vi "LVFunction_Imop_SlopesPostProcessor_Apply Apply Filter.vi"(0 "HasoSlopes in":refnum<class "HasoSlopes.lvclass">, 5 "HasoSlopes OUT":refnum<class "HasoSlopes.lvclass">, 7 "filter":T1, 11 "error in (no error)":errorcluster) -> (4 "HasoSlopes out":refnum<class "HasoSlopes.lvclass">, 6 "HasoSlopes OUT 2":refnum<class "HasoSlopes.lvclass">, 15 "error out":errorcluster)   [LabVIEW 2020]
uses:
  HasoSlopes.lvclass
  SlopesPostProcessorList - Filter.ctl
  LVClass_HasoSlopes Read HasoSlopes _ property.vi
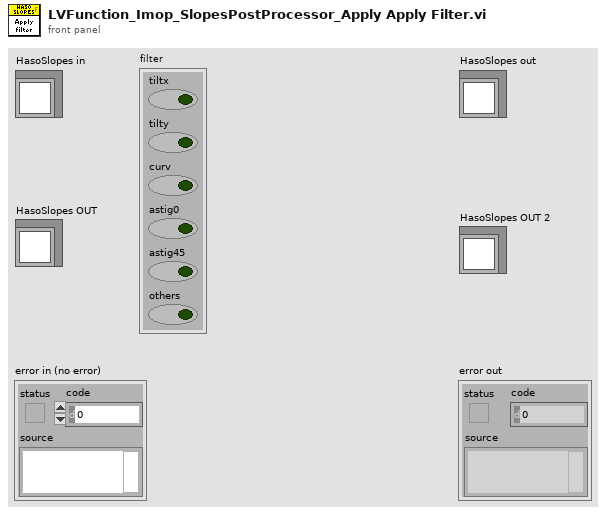
[diagram p1: front panel]
types:
  T1 = typedef "SlopesPostProcessorList - Filter.ctl" = cluster{"tiltx":bool, "tilty":bool, "curv":bool, "astig0":bool, "astig45":bool, "others":bool}
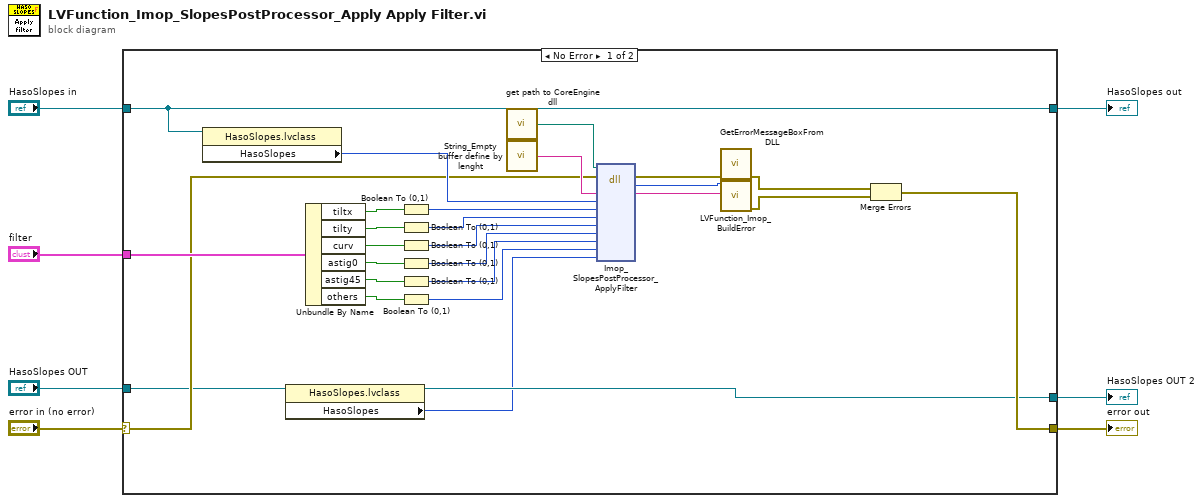
[diagram p0: block diagram]
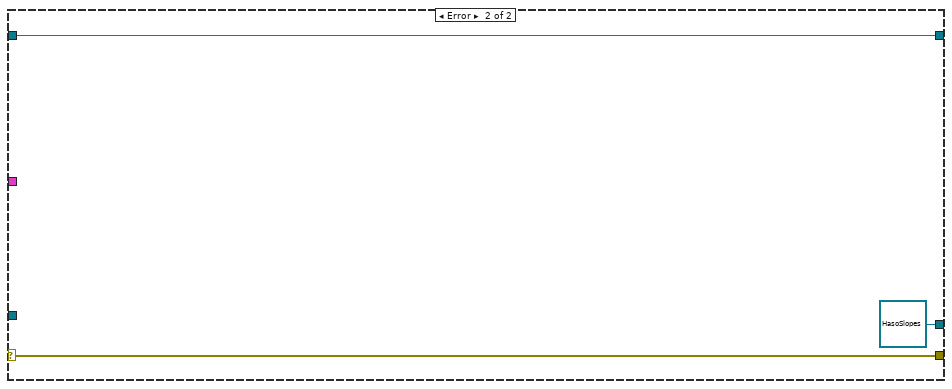
[diagram p2: hidden frame]
diagram:
  n1 = case shown="No Error" "error in (no error)" {
    selector: "error in (no error)" -> [w13 w37]
    tunnel: [w12 w37] -> w3
    tunnel: [w9 w36] -> w4
    tunnel: "HasoSlopes in" -> [w9 w36]
    tunnel: "filter" -> [w14 _]
    tunnel: "HasoSlopes OUT" -> [w11 _]
    tunnel: [w10 refnum<class "HasoSlopes.lvclass"> refnum ("HasoSlopes OUT")] -> w5
    frame No Error {
      n2 = property class="HasoSlopes.lvclass"(reference=w9) -> ("HasoSlopes"=w15:i32)  [unwired: 1 in, 2 out]
      n3 = property class="HasoSlopes.lvclass"(reference=w11) -> (reference out=w10:refnum<class "HasoSlopes.lvclass">, "HasoSlopes"=w8:i32)  [unwired: 1 in, 1 out]
      n4 = Unbundle By Name(w14) -> ("tiltx"=w23:bool, "tilty"=w24:bool, "curv"=w25:bool, "astig0"=w26:bool, "astig45"=w27:bool, "others"=w28:bool)
      n5 = Boolean To (0,1)(Boolean=w23) -> (0, 1=w29:i16)
      n6 = Boolean To (0,1)(Boolean=w24) -> (0, 1=w30:i16)
      n7 = Boolean To (0,1)(Boolean=w25) -> (0, 1=w31:i16)
      n8 = Boolean To (0,1)(Boolean=w26) -> (0, 1=w32:i16)
      n9 = Boolean To (0,1)(Boolean=w27) -> (0, 1=w33:i16)
      n10 = Boolean To (0,1)(Boolean=w28) -> (0, 1=w34:i16)
      n11 = call "get path to CoreEngine dll.vi"() -> ("path to c_interface_vc100.dll"=w16:path)  [unwired: 12 in, 3 out]
      n12 = call "String_Empty buffer define by lenght.vi"() -> ("Empty buffer"=w17:string)  [unwired: 1 in]
      n13 = dll-call lib="D:/FLE/0.Code/CoreEngine4_Suite/LV2011_interface/DLLs/c_interface_vc100.dll" fn="Imop_SlopesPostProcessor_ApplyFilter"(path in=w16, error in=w13, "Message"=w17, "SlopesPostProcessor"=w15, "tiltx"=w29, "tilty"=w30, "curv"=w31, "astig0"=w32, "astig45"=w33, "others"=w34, "HasoSlopes OUT"=w8) -> (error out=w18:errorcluster, "return type"=w19:i32, "Message"=w20:string)  [unwired: 9 in, 1 out]
      n14 = call "GetErrorMessageBoxFromDLL.vi"("error IN"=w18) -> ("error OUT"=w21:errorcluster)  [unwired: 10 in]
      n15 = call "LVFunction_Imop_BuildError.vi"("code"=w19, "String to Prepend to source (\"\")"=w20) -> ("error out"=w22:errorcluster)  [unwired: 13 in]
      n16 = Merge Errors(w21, w22) -> (w12:errorcluster)
    }
    frame Error {
    }
  }
  "error out" <- w3
  "HasoSlopes out" <- w4
  "HasoSlopes OUT 2" <- w5
